vi "Read From Configuration File.vi"(7 "Settings":T1, 8 "error in (no error)":errorcluster) -> (0 "error out":errorcluster, 2 "XML Elements":string)   [LabVIEW 2014]
uses:
  Controls/Configuration Files.ctl
  <vilib>/Utility/xml.llb/Read From XML File(string).vi
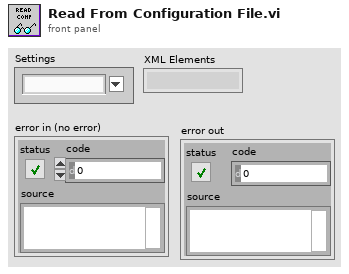
[diagram p1: front panel]
types:
  T1 = typedef "Configuration Files.ctl" = string
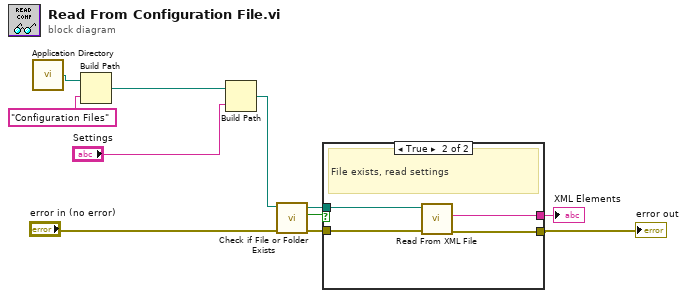
[diagram p0: block diagram]
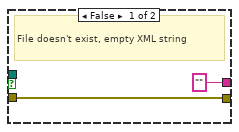
[diagram p2: hidden frame]
diagram:
  n1 = call <vilib>:"Application Directory.vi"() -> ("Application Directory"=w4:path)
  n2 = Build Path(base path=w4, name or relative path="Configuration Files") -> (appended path=w6:path)
  n3 = Build Path(base path=w6, name or relative path="Settings") -> (appended path=w9:path)
  n4 = call <vilib>:"Check if File or Folder Exists.vi"("error in (no error)"="error in (no error)", "path"=w9) -> ("error out"=w7:errorcluster, "file or folder exists?"=w10:bool, "dup path"=w11:path)  [unwired: 7 in]
  n5 = case shown="True" w10 {
    tunnel: w7 -> [w13 w17]
    tunnel: w11 -> [_ w16]
    tunnel: [w13 w15] -> w1
    tunnel: ["" ("XML Elements") w14] -> w2
    frame False {
      # "File doesn't exist, empty XML string"
    }
    frame True {
      # "File exists, read settings"
      n6 = call-poly <vilib>:"Read From XML File.vi"("error in (no error)"=w17, "XML File Path"=w16) -> ("error out"=w15:errorcluster, "XML Elements"=w14:string)  [unwired: 7 in, 1 out]
    }
  }
  "error out" <- w1
  "XML Elements" <- w2
